vi "Dpc Set Spi Mode.vi"(0 "hif":u32, 1 "perc":i32, 5 "idMode":i32, 7 "idDir":i32, 9 "idSpeed":i32, 11 "error in (no error)":errorcluster, 12 "ptrid":u16) -> (3 "perc out":i32, 4 "hif out":u32, 6 "function return":i32, 14 "ptrid out":u16, 15 "error out":errorcluster)   [LabVIEW 2011, in "LVH-Adept.lvlib" / "DPCUTIL.lvlib"]
doc: "DPCAPI BOOL DpcSetSpiMode(HANDLE hif, INT32 idMode, INT32 idDir, INT32 idSpeed, ERC * perc, TRID * ptrid);"
uses:
  DPCUTIL.lvlib
  Resources/dpcutil.dll
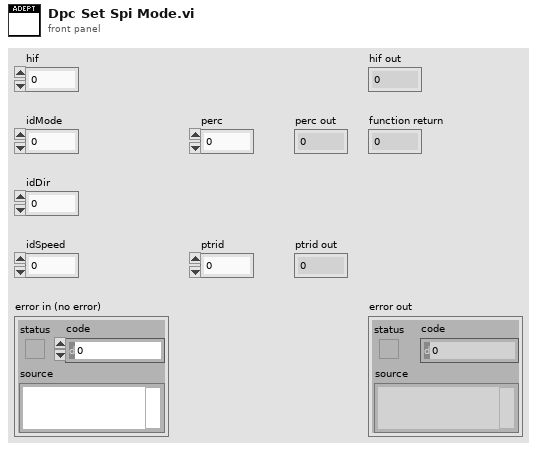
[diagram p1: front panel]
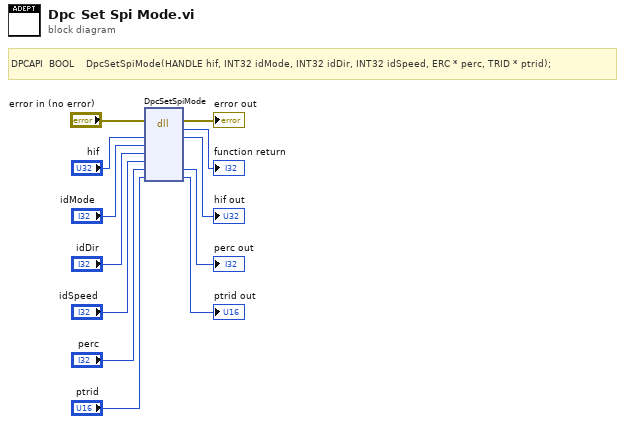
[diagram p0: block diagram]
diagram:
  # "DPCAPI  BOOL    DpcSetSpiMode(HANDLE hif, INT32 idMode, INT32 idDir, INT32 idSpeed, ERC * perc, TRID * ptrid);"
  n1 = dll-call lib="C:/github/labviewhacker/LVH-Adept/LabVIEW/vi.lib/LabVIEW Hacker/Adept/Private/Resources/dpcutil.*" fn="DpcSetSpiMode"(error in="error in (no error)", "hif"="hif", "idMode"="idMode", "idDir"="idDir", "idSpeed"="idSpeed", "perc"="perc", "ptrid"="ptrid") -> (error out=→"error out":errorcluster, →"function return":i32, "hif"=→"hif out":u32, "perc"=→"perc out":i32, "ptrid"=→"ptrid out":u16)  [unwired: 5 in, 1 out]
